vi "VEHICLE_Model.vi"() -> ()   [LabVIEW 2017]
doc: "This example describes how to programmatically call a Model compiled by NI VeriStand and run this model in LabVIEW."
uses:
  <vilib>/Platform/TimedLoop/XDataNode/timing_clust.ctl
  <vilib>/Platform/TimedLoop/XDataNode/nitl_modes.ctl
  <vilib>/Platform/TimedLoop/XDataNode/wakeup.ctl
  <vilib>/Model Interface Toolkit/Model Interface Toolkit.lvclass/Model Interface Toolkit.ctl
  <vilib>/Model Interface Toolkit/Model Update.vi
  <vilib>/Model Interface Toolkit/Tick Model.vi
  <vilib>/Model Interface Toolkit/Probe Signals.vi
  <vilib>/Model Interface Toolkit/Multirate/Dispatch Model Tasks.vi
  <vilib>/Model Interface Toolkit/Call Model Start Routine.vi
  <vilib>/Model Interface Toolkit/Handle Error.vi
  <vilib>/Model Interface Toolkit/Multirate/Wait on Tasks.vi
  <vilib>/FPGAPlugInAG/myRIO-1900/niLvFpga_Open_myRIO-1900.vi
  <vilib>/rvi/interface/common/dynamic/niFpgaDynamicAddResources.vi
  <vilib>/Utility/error.llb/Error Cluster From Error Code.vi
  <vilib>/rvi/errors/niLvFpgaAdjustHostInterfaceError.vi
  <vilib>/Model Interface Toolkit/Check Error.vi
  <vilib>/Model Interface Toolkit/Generate Error Cluster.vi
  <vilib>/Platform/TimedLoop/scheduler/LVUserAPI/Fire Software-Triggered Timing Source.vi
  <vilib>/FPGAPlugInAG/Dynamic/niLvFpga_Close_Dynamic.vi
  <vilib>/Platform/TimedLoop/XDataNode/XDataNode.xnode
  <vilib>/rvi/interface/nirviOpenFPGA/nirviOpenFPGA.xnode
  FPGA Bitfiles/vehiclemyRIO2_FPGATarget_FPGAIO_ha45vdtE-E8.lvbitx
  Fpga_test.vi
  <vilib>/rvi/interface/nirviReadWriteControl/nirviReadWriteControl.xnode
  <vilib>/rvi/interface/nirviCloseFPGA/nirviCloseFPGA.xnode
  <vilib>/Model Interface Toolkit/Model Interface Toolkit.lvclass
  <vilib>/Platform/TimedLoop/XDataNode/XDNodeRunTimeDep.lvlib
  <vilib>/rvi/interface/Simulation/niFpgaSimulationCallBeginRW.vi
  NiFpgaLv.dll
panel:
  in  "Scale u2":dbl=5.0
  in  "Scale u1":dbl=5.0
  in  "Offset u2":dbl=2.0
  in  "Offset u1":dbl=2.0
  in  "Scale x3":dbl=10.0
  in  "Scale x2":dbl=10.0
  in  "Scale x1":dbl=10.0
  in  "Offset x3":dbl=5.0
  in  "Offset x2":dbl
  in  "Offset x1":dbl
  in  "x3_0":dbl
  in  "x2_0":dbl=0.6
  in  "x1_0":dbl=0.6
  out "counter":dbl
  in  "SCOTS timestep":dbl=0.3
  out "u_2":dbl
  out "u_1":dbl
  out "x3":dbl
  out "Execution Time (ms)":u32
  out "Iteration":i32
  in  "Clear Graphs":bool
  out "States":cluster{"x1":dbl[], "y1":dbl[]}[](graph)
  in  "Chart History 2":i32=10000
  in  "Chart History 1":i32=10000
  out "x2":cluster{dbl[], dbl[]}(graph)
  out "x1":cluster{dbl[], dbl[]}(graph)
  in  "Chart History 0":i32=10000
  out "x2":dbl
  out "x1":dbl
  out "Model Period (s)":dbl
  in  "stop":bool
  # "Overview: This test runs in only one MyRIO module. Simulink code is called every 5ms. Outputs and Inputs are sent/received every 0.5s\nRequirements: LabVIEW Model Interface Toolkit\nInstructions:\n1. Connect: AO0 <-> AI0, AO1 <-> AI1, DIO0 <-> DIO1 \n2. Run the FPGA controller code\n3. Specify parameters and run this VI"
  # "INPUTS CONVERSION"
  # "STATES CONVERSION"
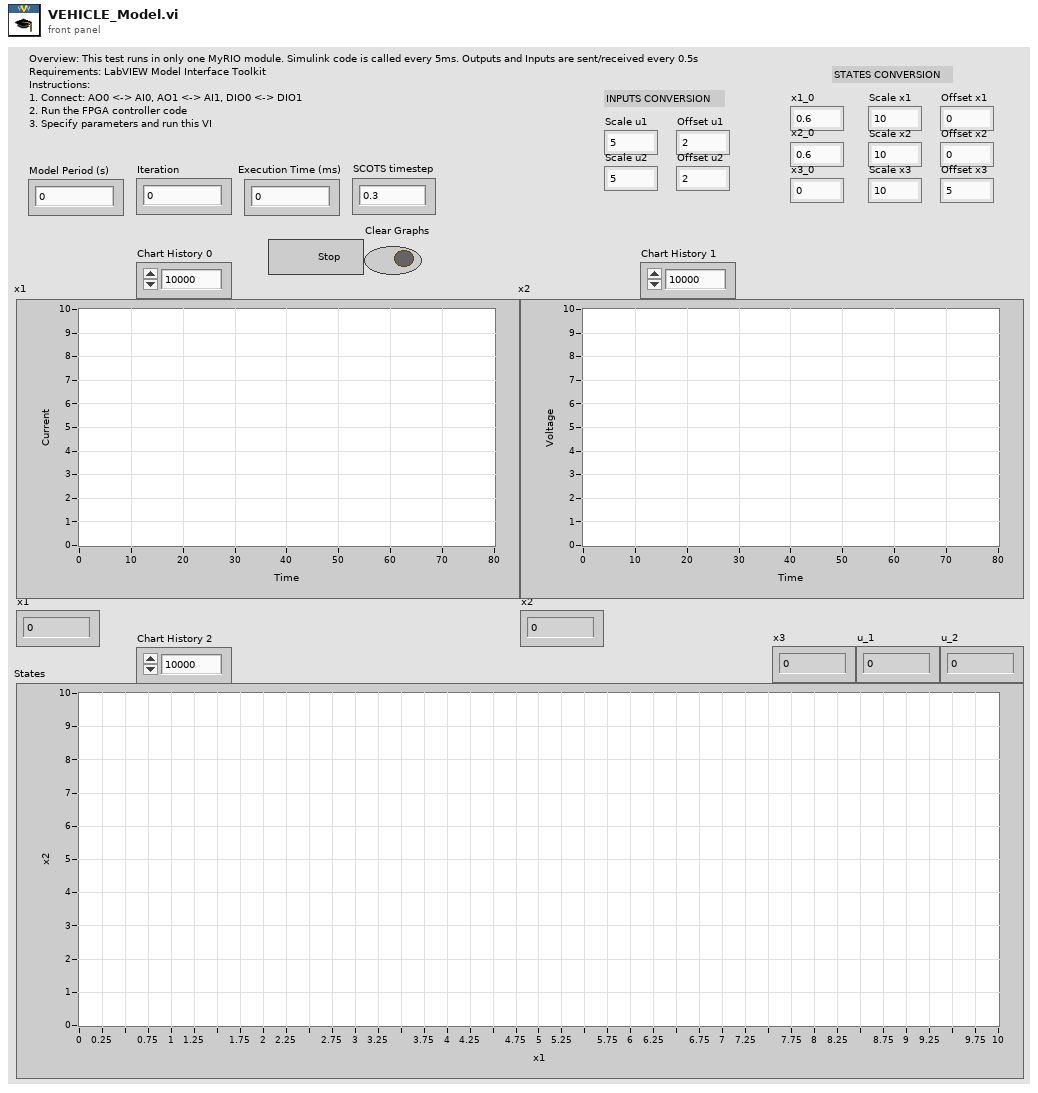
[diagram p1: front panel]
types:
  T1 = typedef "XDNodeRunTimeDep.lvlib/timing_clust.ctl" = cluster{"Expected End [f-1]":u64, "Actual End [f-1]":u64, "Finished Late? [f-1]":bool, "Expected End [i-1]":u64, "Actual End [i-1]":u64, "Finished Late? [i-1]":bool, "Expected Start [i]":u64, "Actual Start [i]":u64, "Expected Start [f]":u64, "Actual Start [f]":u64, "Source Name":string, "Structure Name":string, "Period":i64, "Deadline":i64, "Offset":i64, "Start":i64, "Priority":i32, "Timeout":i32, "Mode":T2, "Wakeup Reason":T3, "Error":errorcluster, "Source Type":string, "Secondary Source Type":string, "Global End Time":u64, "Global Start Time":u64, "Frame Duration":u64, "Iteration Duration":u64, "Assigned CPU":i32, "I/O Scan Engine Mode":u32}
  T2 = typedef "XDNodeRunTimeDep.lvlib/nitl_modes.ctl" = enum32{"No Change", "Process missed periods, maintain original phase", "Discard missed periods, maintain original phase", "Process missed periods, ignore original phase", "Discard missed periods, ignore original phase"}
  T3 = typedef "XDNodeRunTimeDep.lvlib/wakeup.ctl" = enum32{"Normal", "Aborted", "Asynchronous wakeup", "Timing source error", "Timed loop error", "Timeout"}
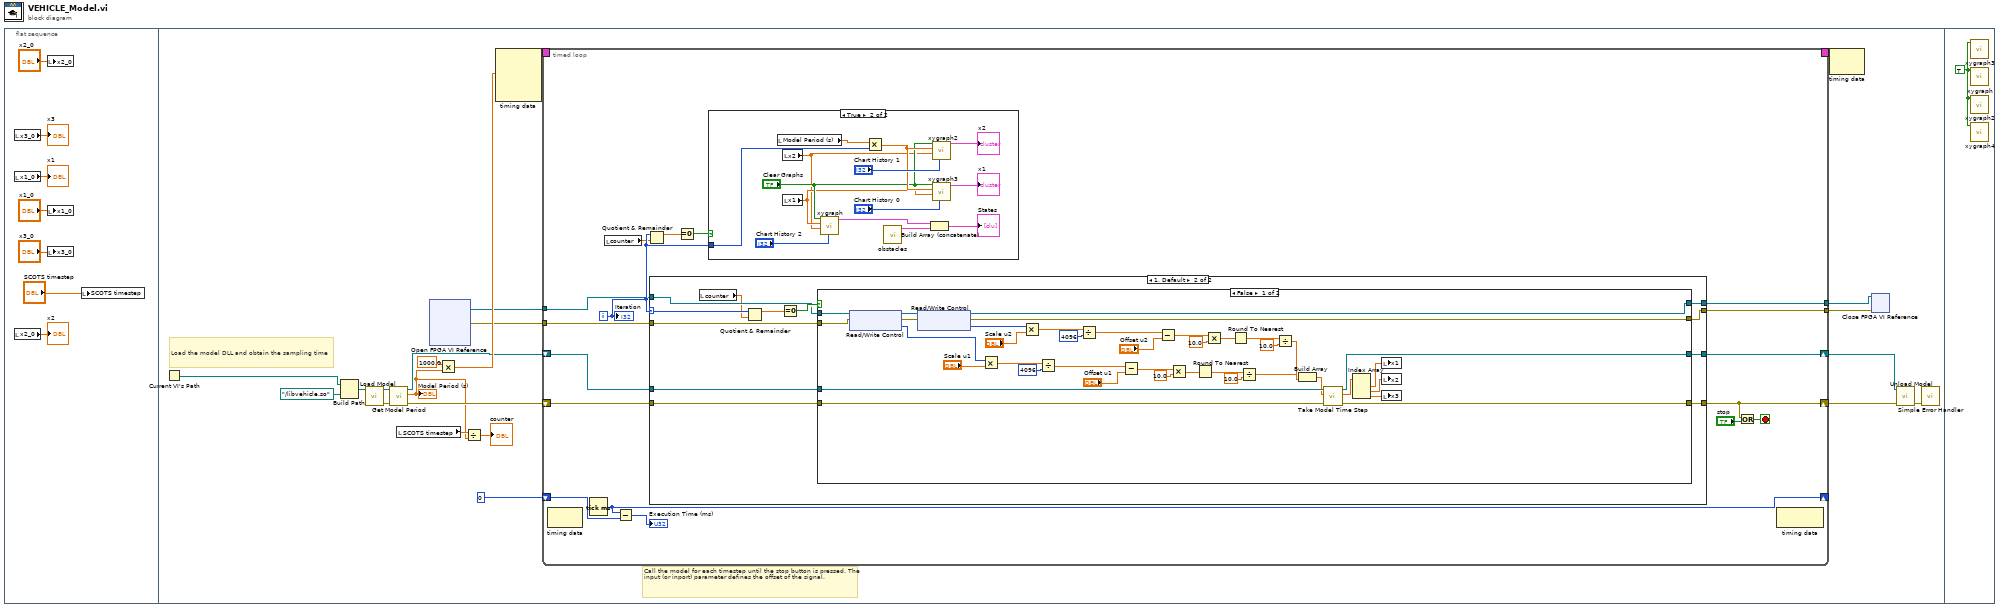
[diagram p0: block diagram]
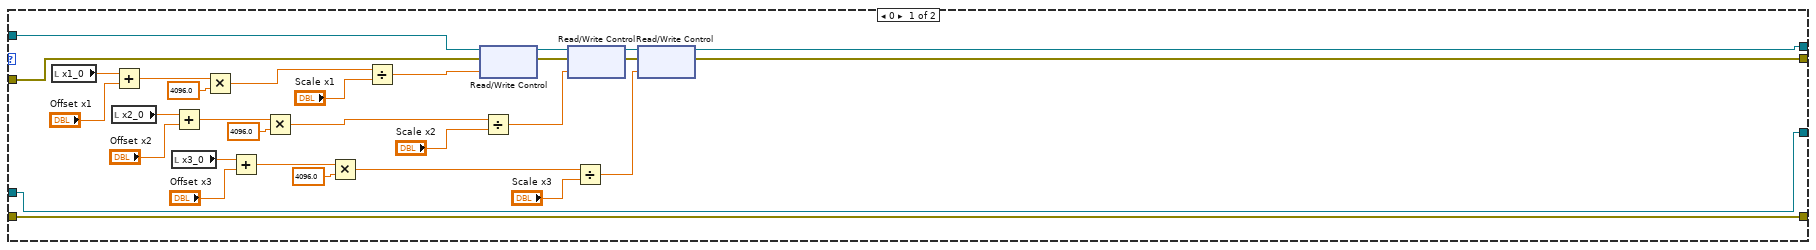
[diagram p3: hidden frame]
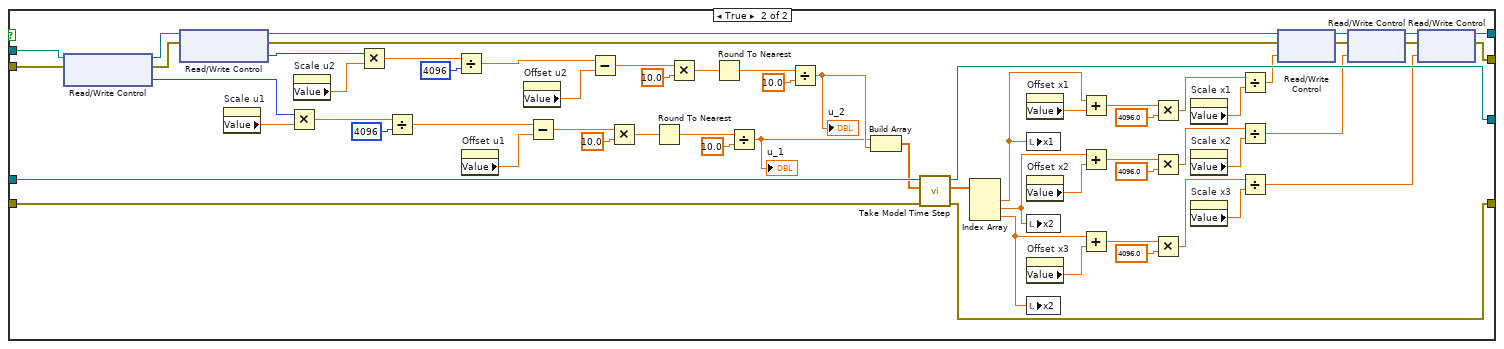
[diagram p4: hidden frame]
diagram:
  n1 = flat-sequence {
    frame #0 {
      n2 = local read "x3_0"() -> (→"x3":dbl)
      n3 = local read "x1_0"() -> (→"x1":dbl)
      n4 = local read "x2_0"() -> (→"x2":dbl)
      n5 = local write "x2_0"("x2_0") -> ()
      n6 = local write "x1_0"("x1_0") -> ()
      n7 = local write "x3_0"("x3_0") -> ()
      n8 = local write "SCOTS timestep"("SCOTS timestep") -> ()
    }
    frame #1 {
      # "Call the model for each timestep until the stop button is pressed. The input (or inport) parameter defines the offset of the signal."
      # "Load the model DLL and obtain the sampling time"
      n9 = Current VI's Path() -> (path=w26:path)
      n10 = Build Path(base path=w26, name or relative path=path "../libvehicle.so" ("Model Path")) -> (appended path=w27:path)
      n11 = call <vilib>:"Load Model.vi"("Model Path"=w27) -> ("error out"=w24:errorcluster, "Model out"=w18:refnum<class "Model Interface Toolkit.lvclass">)  [unwired: 9 in]
      n12 = call <vilib>:"Get Model Period.vi"("error in"=w24, "Model in"=w18) -> ("error out"=w20:errorcluster, "Model Period (s)"=w8:dbl, "Model out"=w22:refnum<class "Model Interface Toolkit.lvclass">)  [unwired: 7 in]
      "Model Period (s)" <- w8
      n13 = local read "SCOTS timestep"() -> (w9:dbl)
      n14 = xnode "Open FPGA VI Reference"() -> ("FPGA VI Reference Out"=w14:refnum<k20>, "error out"=w13:errorcluster)  [unwired: 2 in]
      n15 = Multiply(x=1000.0, y=w8) -> (x*y=w23:dbl)
      n16 = Divide(x=w9, y=w8) -> (x/y=→"counter":dbl)
      n17 = node-c288(w23) -> (w29:T1)  [unwired: 3 in]
      n18 = timed-loop {
        timing: w29 -> [_]
        timing-out: [_] -> w28
        shift-right: [w45] -> w21
        shift-left: w22 -> [w46]
        shift-right: [w41] -> w19
        shift-left: w20 -> [w44]
        shift-right: [w38] -> _
        shift-left: 0 -> [w37]
        tunnel: w14 -> [w34]
        tunnel: w13 -> [w31]
        tunnel: [w33] -> w12
        tunnel: [w32] -> w11
        i -> [w36]
        stop <- w42 stop-if-true
        n19 = node-c288() -> ()  [unwired: 1 in, 1 out]
        n20 = Tick Count (ms)() -> (millisecond timer value=w38:u32)
        n21 = local read "counter"() -> (w30:dbl)
        n22 = Subtract(x=w38, y=w37) -> (x-y=→"Execution Time (ms)":u32)
        n23 = Quotient & Remainder(x=w36, y=w30) -> (x-y*floor(x/y)=w40:dbl)  [unwired: 1 out]
        n24 = case shown="1, Default" w36 {
          selector: w36 -> [_ w97]
          tunnel: w46 -> [w91 w103]
          tunnel: [w91 w101] -> w45
          tunnel: w44 -> [w90 w100]
          tunnel: [w90 w102] -> w41
          tunnel: w34 -> [w87 w96]
          tunnel: [w74 w95] -> w33
          tunnel: [w73 w94] -> w32
          tunnel: w31 -> [w86 w93]
          frame 0 {
            n25 = local read "x1_0"() -> (w64:dbl)
            n26 = local read "x2_0"() -> (w62:dbl)
            n27 = Add(x=w64, y="Offset x1") -> (x+y=w66:dbl)
            n28 = local read "x3_0"() -> (w71:dbl)
            n29 = Add(x=w62, y="Offset x2") -> (x+y=w63:dbl)
            n30 = Multiply(x=w66, y=sgl 4096.0 ("Slide")) -> (x*y=w83:dbl)
            n31 = Add(x=w71, y="Offset x3") -> (x+y=w72:dbl)
            n32 = Multiply(x=w63, y=sgl 4096.0 ("Slide")) -> (x*y=w81:dbl)
            n33 = Multiply(x=w72, y=sgl 4096.0 ("Slide")) -> (x*y=w79:dbl)
            n34 = Divide(x=w83, y="Scale x1") -> (x/y=w75:dbl)
            n35 = xnode "Read/Write Control"("FPGA VI Reference In"=w87, "error in"=w86, "x1_read"=w75) -> ("FPGA VI Reference Out"=w89:refnum<k20>, "error out"=w85:errorcluster)
            n36 = Divide(x=w81, y="Scale x2") -> (x/y=w76:dbl)
            n37 = xnode "Read/Write Control"("FPGA VI Reference In"=w89, "error in"=w85, "x2_read"=w76) -> ("FPGA VI Reference Out"=w88:refnum<k20>, "error out"=w84:errorcluster)
            n38 = Divide(x=w79, y="Scale x3") -> (x/y=w77:dbl)
            n39 = xnode "Read/Write Control"("FPGA VI Reference In"=w88, "error in"=w84, "x3_read"=w77) -> ("FPGA VI Reference Out"=w74:refnum<k20>, "error out"=w73:errorcluster)
          }
          frame 1, Default {
            n40 = local read "counter"() -> (w92:dbl)
            n41 = Quotient & Remainder(x=w97, y=w92) -> (x-y*floor(x/y)=w98:dbl)  [unwired: 1 out]
            n42 = Equal To 0?(x=w98) -> (x = 0?=w99:bool)
            n43 = case shown="False" w99 {
              tunnel: w103 -> [w142 w204]
              tunnel: [w140 w203] -> w102
              tunnel: [w141 w202] -> w101
              tunnel: w100 -> [w139 w201]
              tunnel: w96 -> [w137 w180]
              tunnel: [w126 w197] -> w95
              tunnel: [w124 w196] -> w94
              tunnel: w93 -> [w136 w175]
              frame False {
                n44 = xnode "Read/Write Control"("FPGA VI Reference In"=w137, "error in"=w136) -> ("FPGA VI Reference Out"=w127:refnum<k20>, "error out"=w125:errorcluster, "output1_read"=w135:u16)
                n45 = xnode "Read/Write Control"("FPGA VI Reference In"=w127, "error in"=w125) -> ("FPGA VI Reference Out"=w126:refnum<k20>, "error out"=w124:errorcluster, "output2_read"=w128:u16)
                n46 = Multiply(x=w135, y="Scale u1") -> (x*y=w134:dbl)
                n47 = Multiply(x=w128, y="Scale u2") -> (x*y=w131:dbl)
                n48 = Divide(x=w134, y=u16 4096) -> (x/y=w132:dbl)
                n49 = Divide(x=w131, y=u16 4096) -> (x/y=w129:dbl)
                n50 = Subtract(x=w132, y="Offset u1") -> (x-y=w107:dbl)
                n51 = Subtract(x=w129, y="Offset u2") -> (x-y=w112:dbl)
                n52 = Multiply(x=w107, y=10.0) -> (x*y=w109:dbl)
                n53 = Round To Nearest(number=w109) -> (nearest integer value=w105:dbl)
                n54 = Multiply(x=w112, y=10.0) -> (x*y=w114:dbl)
                n55 = Round To Nearest(number=w114) -> (nearest integer value=w104:dbl)
                n56 = Divide(x=w105, y=10.0) -> (x/y=w106:dbl)
                n57 = Divide(x=w104, y=10.0) -> (x/y=w111:dbl)
                n58 = Build Array(w106, w111) -> (w138:dbl[])
                n59 = call <vilib>:"Take Model Time Step.vi"("error in (no error)"=w139, "Inport Array"=w138, "Model in"=w142) -> ("error out"=w140:errorcluster, "Outport Array out"=w119:dbl[], "Model out"=w141:refnum<class "Model Interface Toolkit.lvclass">)  [unwired: 6 in]
                n60 = Index Array(array=w119) -> (element #1=w118:dbl, element #2=w117:dbl, element #3=w116:dbl)  [unwired: 3 in]
                n61 = local write "x1"(w118) -> ()
                n62 = local write "x2"(w117) -> ()
                n63 = local write "x3"(w116) -> ()
              }
              frame True {
                n64 = xnode "Read/Write Control"("FPGA VI Reference In"=w180, "error in"=w175) -> ("FPGA VI Reference Out"=w179:refnum<k20>, "error out"=w176:errorcluster, "output1_read"=w184:u16)
                n65 = xnode "Read/Write Control"("FPGA VI Reference In"=w179, "error in"=w176) -> ("FPGA VI Reference Out"=w177:refnum<k20>, "error out"=w178:errorcluster, "output2_read"=w171:u16)
                n66 = property on="Scale u1" class="DigNum (strict)"() -> ("Value"=w157:dbl)  [unwired: 2 in, 2 out]
                n67 = Multiply(x=w184, y=w157) -> (x*y=w183:dbl)
                n68 = property on="Scale u2" class="DigNum (strict)"() -> ("Value"=w158:dbl)  [unwired: 2 in, 2 out]
                n69 = Multiply(x=w171, y=w158) -> (x*y=w174:dbl)
                n70 = Divide(x=w183, y=u16 4096) -> (x/y=w181:dbl)
                n71 = Divide(x=w174, y=u16 4096) -> (x/y=w172:dbl)
                n72 = property on="Offset u1" class="DigNum (strict)"() -> ("Value"=w156:dbl)  [unwired: 2 in, 2 out]
                n73 = property on="Offset u2" class="DigNum (strict)"() -> ("Value"=w159:dbl)  [unwired: 2 in, 2 out]
                n74 = Subtract(x=w181, y=w156) -> (x-y=w145:dbl)
                n75 = Subtract(x=w172, y=w159) -> (x-y=w154:dbl)
                n76 = Multiply(x=w145, y=10.0) -> (x*y=w147:dbl)
                n77 = Round To Nearest(number=w147) -> (nearest integer value=w143:dbl)
                n78 = Multiply(x=w154, y=10.0) -> (x*y=w152:dbl)
                n79 = Round To Nearest(number=w152) -> (nearest integer value=w151:dbl)
                n80 = Divide(x=w143, y=10.0) -> (x/y=w144:dbl)
                "u_1" <- w144
                n81 = Divide(x=w151, y=10.0) -> (x/y=w149:dbl)
                "u_2" <- w149
                n82 = Build Array(w144, w149) -> (w200:dbl[])
                n83 = call <vilib>:"Take Model Time Step.vi"("error in (no error)"=w201, "Inport Array"=w200, "Model in"=w204) -> ("error out"=w203:errorcluster, "Outport Array out"=w205:dbl[], "Model out"=w202:refnum<class "Model Interface Toolkit.lvclass">)  [unwired: 6 in]
                n84 = Index Array(array=w205) -> (element #1=w161:dbl, element #2=w160:dbl, element #3=w155:dbl)  [unwired: 3 in]
                n85 = property on="Offset x1" class="DigNum (strict)"() -> ("Value"=w165:dbl)  [unwired: 2 in, 2 out]
                n86 = local write "x1"(w161) -> ()
                n87 = property on="Offset x2" class="DigNum (strict)"() -> ("Value"=w164:dbl)  [unwired: 2 in, 2 out]
                n88 = local write "x2"(w160) -> ()
                n89 = property on="Offset x3" class="DigNum (strict)"() -> ("Value"=w166:dbl)  [unwired: 2 in, 2 out]
                n90 = local write "x2"(w155) -> ()
                n91 = Add(x=w161, y=w165) -> (x+y=w162:dbl)
                n92 = Add(x=w160, y=w164) -> (x+y=w163:dbl)
                n93 = Add(x=w155, y=w166) -> (x+y=w170:dbl)
                n94 = Multiply(x=w162, y=sgl 4096.0 ("Slide")) -> (x*y=w193:dbl)
                n95 = Multiply(x=w163, y=sgl 4096.0 ("Slide")) -> (x*y=w191:dbl)
                n96 = Multiply(x=w170, y=sgl 4096.0 ("Slide")) -> (x*y=w189:dbl)
                n97 = property on="Scale x1" class="DigNum (strict)"() -> ("Value"=w167:dbl)  [unwired: 2 in, 2 out]
                n98 = property on="Scale x2" class="DigNum (strict)"() -> ("Value"=w169:dbl)  [unwired: 2 in, 2 out]
                n99 = property on="Scale x3" class="DigNum (strict)"() -> ("Value"=w168:dbl)  [unwired: 2 in, 2 out]
                n100 = Divide(x=w193, y=w167) -> (x/y=w185:dbl)
                n101 = Divide(x=w191, y=w169) -> (x/y=w186:dbl)
                n102 = Divide(x=w189, y=w168) -> (x/y=w187:dbl)
                n103 = xnode "Read/Write Control"("FPGA VI Reference In"=w177, "error in"=w178, "x1_read"=w185) -> ("FPGA VI Reference Out"=w199:refnum<k20>, "error out"=w194:errorcluster)
                n104 = xnode "Read/Write Control"("FPGA VI Reference In"=w199, "error in"=w194, "x2_read"=w186) -> ("FPGA VI Reference Out"=w198:refnum<k20>, "error out"=w195:errorcluster)
                n105 = xnode "Read/Write Control"("FPGA VI Reference In"=w198, "error in"=w195, "x3_read"=w187) -> ("FPGA VI Reference Out"=w197:refnum<k20>, "error out"=w196:errorcluster)
              }
            }
          }
        }
        n106 = Equal To 0?(x=w40) -> (x = 0?=w39:bool)
        n107 = case shown="True" w39 {
          tunnel: w36 -> [_ w53]
          frame False {
          }
          frame True {
            n108 = local read "Model Period (s)"() -> (w49:dbl)
            n109 = local read "x2"() -> (w47:dbl)
            n110 = local read "x1"() -> (w48:dbl)
            n111 = call "xygraph.vi"("Chart History (10,000)"="Chart History 2", "Y Value"=w47, "X Value"=w48, "clear 1"="Clear Graphs") -> ("Cluster"=w55:cluster{dbl[], dbl[]})  [unwired: 7 in]
            n112 = Multiply(x=w49, y=w53) -> (x*y=w52:dbl)
            n113 = call "obstacles.vi"() -> ("appended array"=w50:cluster{"x1":dbl[], "y1":dbl[]}[])  [unwired: 10 in]
            n114 = Build Array (concatenate)(w55, w50) -> (→"States":cluster{"x1":dbl[], "y1":dbl[]}[])
            n115 = call "xygraph2.vi"("Chart History (10,000)"="Chart History 1", "Y Value"=w47, "X Value"=w52, "clear 2"="Clear Graphs") -> ("Cluster"=→"x2":cluster{dbl[], dbl[]})  [unwired: 7 in]
            n116 = call "xygraph3.vi"("Chart History (10,000)"="Chart History 0", "Y Value"=w48, "X Value"=w52, "clear"="Clear Graphs") -> ("Cluster"=→"x1":cluster{dbl[], dbl[]})  [unwired: 7 in]
          }
        }
        n117 = Or(x=w41, y="stop") -> (x .or. y?=w42:bool)
        n118 = node-c288() -> ()  [unwired: 1 in, 1 out]
        "Iteration" <- w36
      }
      n119 = node-c288(w28) -> ()  [unwired: 1 out]
      n120 = xnode "Close FPGA VI Reference"("FPGA VI Reference In"=w12, "error in"=w11) -> ()  [unwired: 1 out]
      n121 = call <vilib>:"Unload Model.vi"("error in (no error)"=w19, "Model in"=w21) -> ("error out"=w17:errorcluster)  [unwired: 9 in]
      n122 = call <vilib>:"Simple Error Handler.vi"("error in (no error)"=w17) -> ()  [unwired: 4 in, 5 out]
    }
    frame #2 {
      w212 = TRUE
      n123 = call "xygraph3.vi"("clear"=w212) -> ()  [unwired: 10 in, 1 out]
      n124 = call "xygraph.vi"("clear 1"=w212) -> ()  [unwired: 10 in, 1 out]
      n125 = call "xygraph2.vi"("clear 2"=w212) -> ()  [unwired: 10 in, 1 out]
      n126 = call "xygraph4.vi"("clear"=w212) -> ()  [unwired: 10 in, 1 out]
    }
  }
